vi "Get OD Index.vi"(8 "error in (no error)":errorcluster, 11 "PDO Communication Parameter in":refnum<class "PDO Communication Parameter.lvclass">) -> (0 "error out":errorcluster, 2 "OD Index":u16 format="%.0x", 3 "PDO Communication Parameter out":refnum<class "PDO Communication Parameter.lvclass">)   [LabVIEW 2019, in "PDO Grid.lvlib" / "PDO Communication Parameter.lvclass"]
uses:
  PDO Communication Parameter.lvclass
  PDO Communication Parameter.lvclass/PDO Communication Parameter.ctl
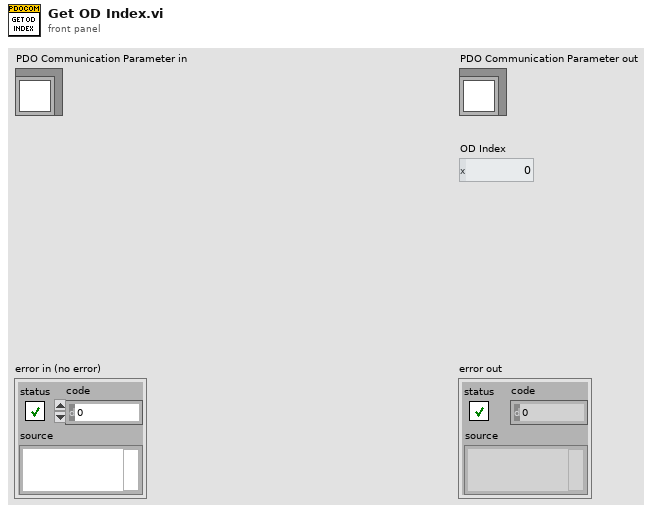
[diagram p1: front panel]
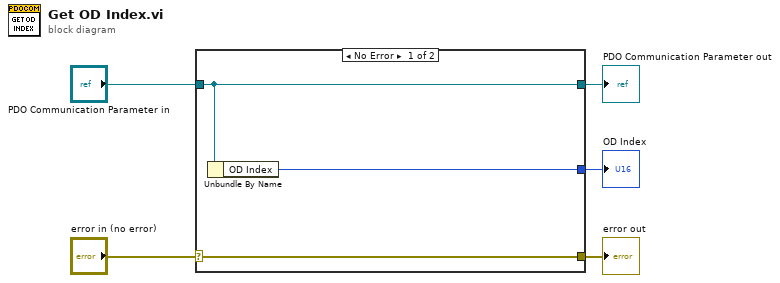
[diagram p0: block diagram]
diagram:
  n1 = case shown="No Error" "error in (no error)" {
    selector: "error in (no error)" -> [w8 w9]
    tunnel: [w8 w9] -> w4
    tunnel: [w7 w10] -> w2
    tunnel: "PDO Communication Parameter in" -> [w7 w10]
    tunnel: [w6 _] -> w1
    frame No Error {
      n2 = Unbundle By Name(w7) -> ("OD Index"=w6:u16)
    }
    frame Error {
    }
  }
  "error out" <- w4
  "PDO Communication Parameter out" <- w2
  "OD Index" <- w1
